vi "Identify.vi"(8 "error in (no error)":errorcluster, 11 "Factory Plugin Framework in":refnum<class "Factory Plugin Framework.lvclass">) -> (0 "error out":errorcluster, 2 "Plugin is Valid":bool, 3 "Factory Plugin Framework out":refnum<class "Factory Plugin Framework.lvclass">)   [LabVIEW 2016, in "Factory Plugin Framework.lvlib" / "Factory Plugin Framework.lvclass"]
uses:
  Factory Plugin Framework.lvclass
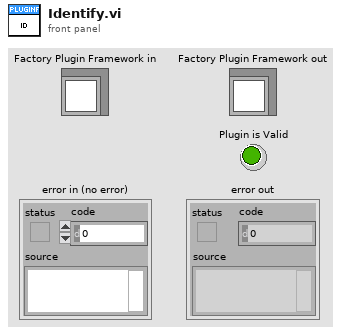
[diagram p1: front panel]
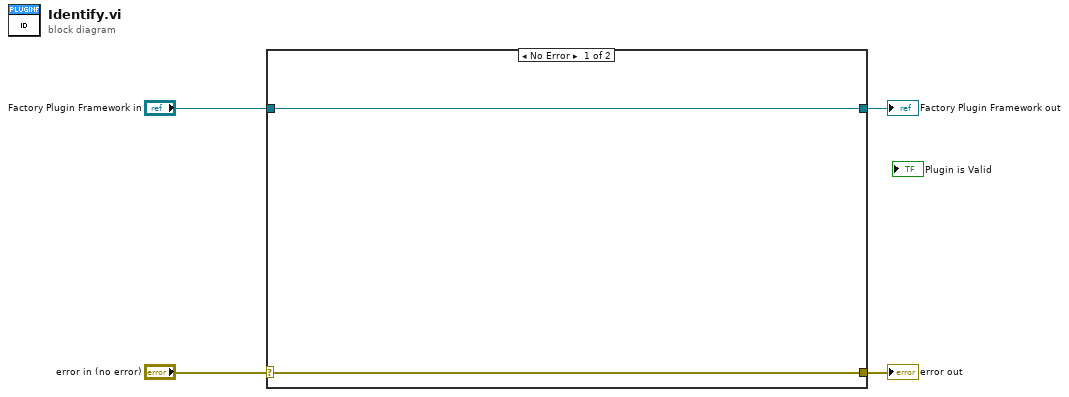
[diagram p0: block diagram]
diagram:
  n1 = case shown="No Error" "error in (no error)" {
    selector: "error in (no error)" -> [w5 w8]
    tunnel: [w5 w8] -> w3
    tunnel: [w6 w7] -> w1
    tunnel: "Factory Plugin Framework in" -> [w6 w7]
    frame No Error {
    }
    frame Error {
    }
  }
  "error out" <- w3
  "Factory Plugin Framework out" <- w1
